vi "Verify Acoustic Calibration.vi"(0 "TSM context":T1, 5 "Cal File Path":path, 7 "Frequency - dBSPL":cluster{"Frequency (Hz)":dbl, "dB SPL":dbl}[](array[cluster])) -> (4 "Per-Site Per-FreqAmpPair dB SPL":dbl[][](array[numeric]), 15 "error out":errorcluster)   [LabVIEW 2020]
doc: "Verifies the calibration data saved in the Cal File. An array of amplitude values is obtained from the Cal file for the respective Freq-dB SPL list passed by the user. Then, a sweep is performed for Freq-Amp pair to obtain back dB SPL to calculate the Error delta (in dB SPL) which is later published to TS layer for Limit checking."
uses:
  <vilib>/NI_TestStand_SemiconductorModule/NI_TestStand_Semiconductor_Module.lvlibp/PinMap/General/SemiconductorModuleContext.ctl
  SubVIs/Per Site Sweep Data.ctl
  45f10d7d-5394-4cb1-bdbe-9d468bbd36f7.vi
  <vilib>/gmath/interp.llb/Interpolate 2D.vi
  <vilib>/gmath/interp.llb/Interpolate 2D (1d xi,yi).vi
  <vilib>/Utility/error.llb/Error Cluster From Error Code.vi
  <vilib>/NI_TestStand_SemiconductorModule/NI_TestStand_Semiconductor_Module.lvlibp/PinMap/General/Publish/PublishDataDoubleFunctionalTest.vi
  <vilib>/NI_TestStand_SemiconductorModule/NI_TestStand_Semiconductor_Module.lvlibp
panel:
  # "Test conditions ----->"
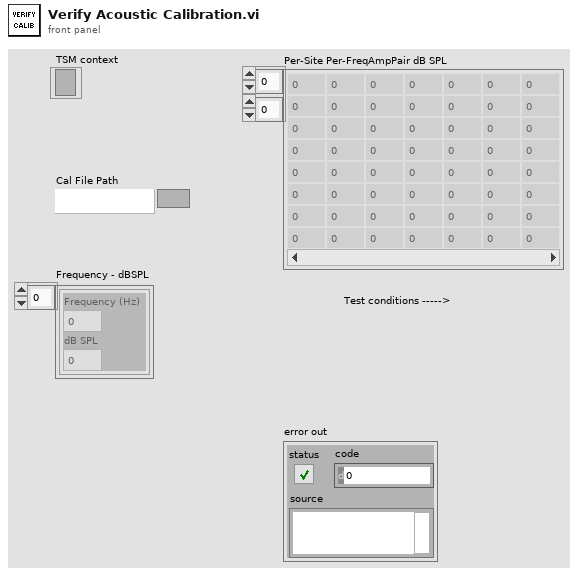
[diagram p1: front panel]
types:
  T1 = typedef "NI_TestStand_Semiconductor_Module.lvlibp/SemiconductorModuleContext.ctl" = refnum<k7>
  T2 = cluster{"TSM context":T1, "Site Numbers":i32[], "Cal File Path":path, "Sampling Rate":dbl, "Frequency - dBSPL List":cluster{"Frequency (Hz)":dbl, "dB SPL":dbl}[], "Per-Site Per-FreqAmpPair dB SPL":dbl[][]}
  T3 = typedef "Per Site Sweep Data.ctl" = cluster{"Site Number":i32, "Frequencies (Hz)":dbl[], "Amplitudes (V)":dbl[]}
  T4 = typedef "Acoustic Cal Data Cluster.ctl" = cluster{"Site Number":i32, "Serial Number":u32, "Ref Mic Sensitivity":dbl, "SPL Axis":dbl[], "Frequency Axis":dbl[], "Speaker Vp":dbl[][], "Ref Mic Cal File Data":string[][], "Speaker Vp Axis":dbl[], "SPL Measurements":dbl[][]}
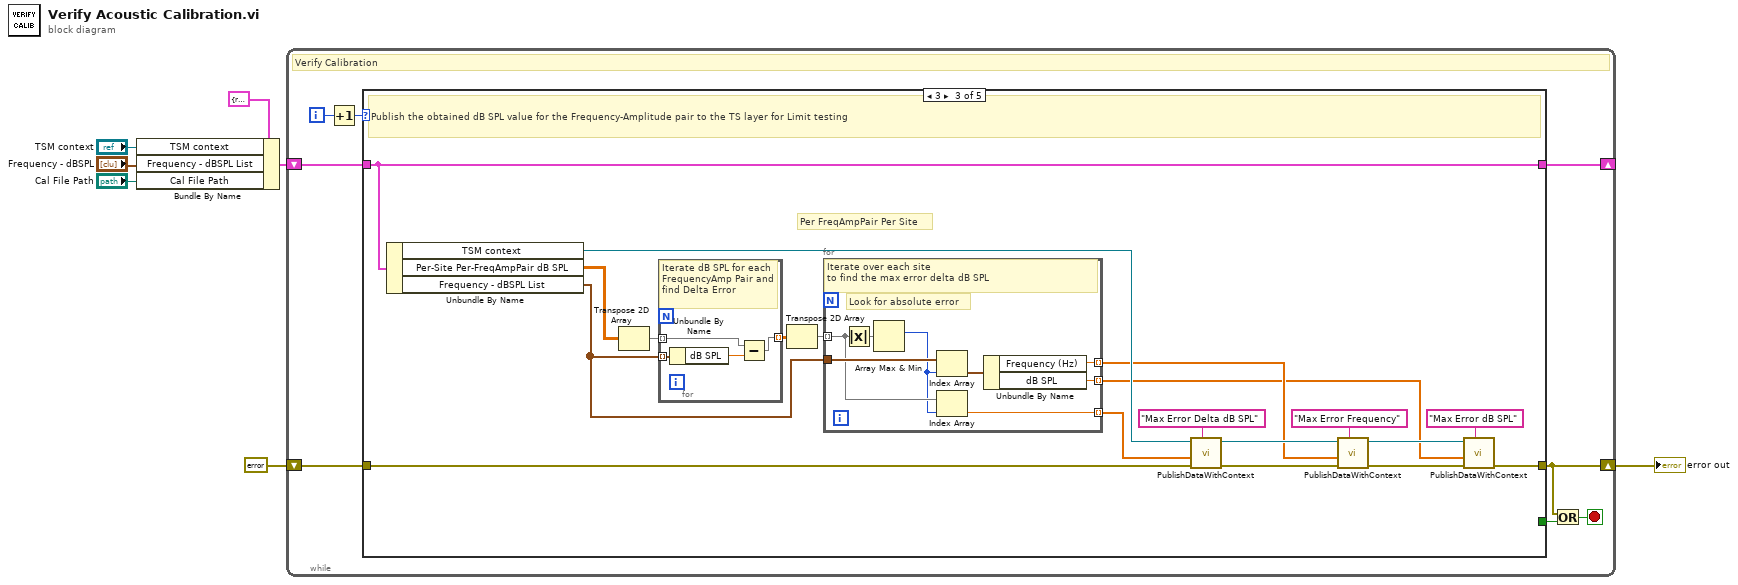
[diagram p0: block diagram]
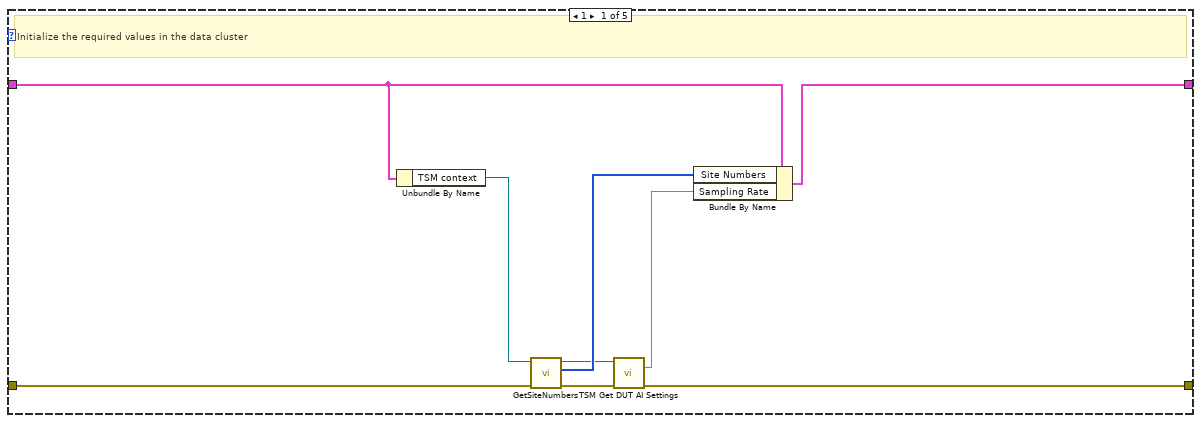
[diagram p2: hidden frame]
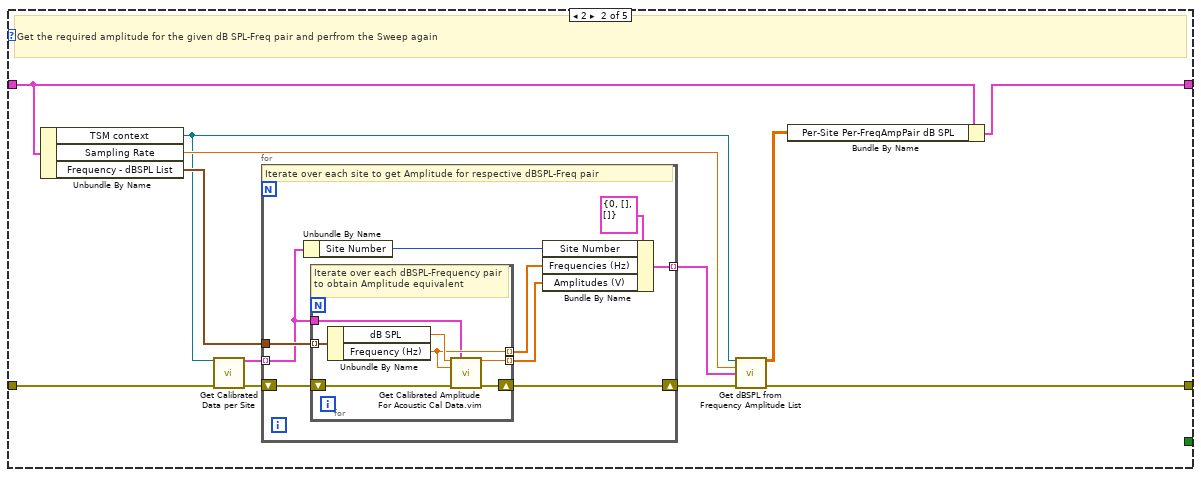
[diagram p3: hidden frame]
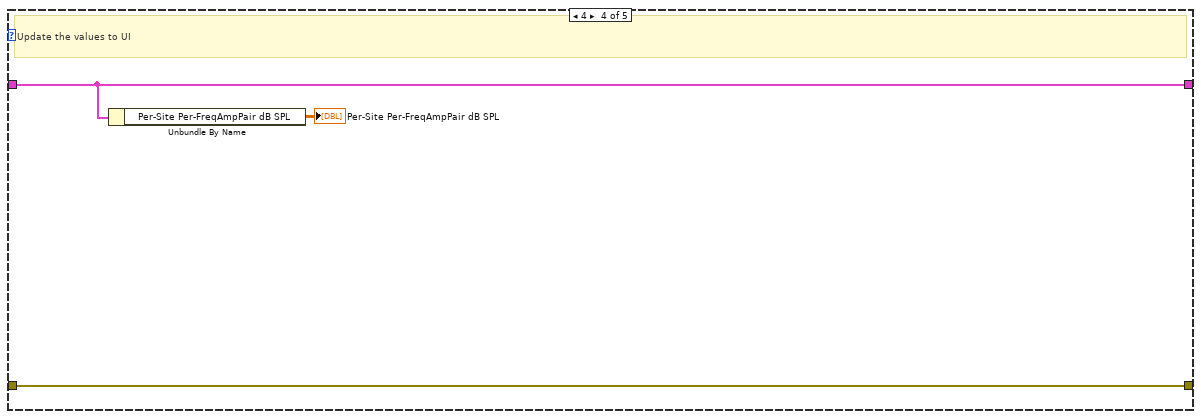
[diagram p4: hidden frame]
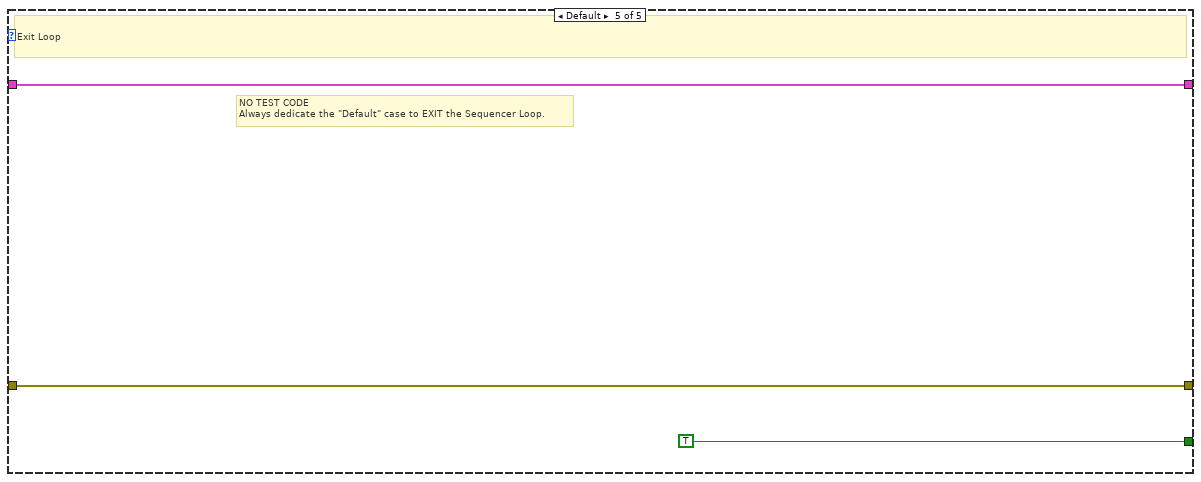
[diagram p5: hidden frame]
diagram:
  n1 = Bundle By Name(cluster=T2 {"TSM context"=refnum, "Site Numbers"=[], "Cal File Path"=path "", "Sampling Rate"=0.0, "Frequency - dBSPL List"=[], "Per-Site Per-FreqAmpPair dB SPL"=[]}, "TSM context"="TSM context", "Frequency - dBSPL List"="Frequency - dBSPL", "Cal File Path"="Cal File Path") -> (w4:T2)
  n2 = while {
    shift-right: [w8] -> w7
    shift-left: errorcluster {"status"=FALSE, "code"=0, "source"=""} ("error in") -> [w14]
    shift-right: [w10] -> _
    shift-left: w4 -> [w11]
    i -> [w15]
    stop <- w9 stop-if-true
    # "Verify Calibration"
    n3 = Increment(x=w15) -> (x+1=w13:i32)
    n4 = case shown="3" w13 {
      tunnel: [w18 w33 w53 w86 w88] -> w8
      tunnel: w14 -> [w17 w28 w65 w86 w88]
      tunnel: [_ _ _ _ TRUE] -> w12
      tunnel: w11 -> [w24 w36 w71 w85 w87]
      tunnel: [w22 w32 w71 w85 w87] -> w10
      frame 1 {
        # "Initialize the required values in the data cluster"
        n5 = Unbundle By Name(w24) -> ("TSM context"=w23:T1)
        n6 = call <vilib>:"GetSiteNumbers.vi"("error in (no error)"=w17, "Semiconductor Module Context"=w23) -> ("error out"=w16:errorcluster, "Site Numbers"=w21:i32[], "Semiconductor Module Context Out"=w20:T1)  [unwired: 6 in, 1 out]
        n7 = call "TSM Get DUT AI Settings.vi"("TSM context"=w20, "error in (no error)"=w16) -> ("Sampling Rate (Hz)"=w19:dbl, "error out"=w18:errorcluster)  [unwired: 9 in, 3 out]
        n8 = Bundle By Name(cluster=w24, "Site Numbers"=w21, "Sampling Rate"=w19) -> (w22:T2)
      }
      frame 2 {
        # "Get the required amplitude for the given dB SPL-Freq pair and perfrom the Sweep again"
        n9 = Unbundle By Name(w36) -> ("TSM context"=w27:T1, "Sampling Rate"=w35:dbl, "Frequency - dBSPL List"=w29:cluster{"Frequency (Hz)":dbl, "dB SPL":dbl}[])
        n10 = call "Get Calibrated Data per Site.vi"("TSM context"=w27, "error in (no error)"=w28) -> ("Per Site Acoustic Cal Data"=w25:T4[], "error out"=w26:errorcluster)  [unwired: 11 in, 1 out]
        n11 = for {
          shift-right: [w45] -> w34
          shift-left: w26 -> [w39]
          tunnel: w29 -> [w44]
          tunnel: [w40] -> w30 mode=indexing
          tunnel: w25 -> [w38] mode=indexing
          # "Iterate over each site to get Amplitude for respective dBSPL-Freq pair"
          n12 = Unbundle By Name(w38) -> ("Site Number"=w37:i32)
          n13 = for {
            shift-right: [w51] -> w45
            shift-left: w39 -> [w52]
            tunnel: w44 -> [w50] mode=indexing
            tunnel: [w48] -> w41 mode=indexing
            tunnel: [w47] -> w42 mode=indexing
            tunnel: w38 -> [w46]
            # "Iterate over each dBSPL-Frequency pair to obtain Amplitude equivalent"
            n14 = Unbundle By Name(w50) -> ("dB SPL"=w49:dbl, "Frequency (Hz)"=w47:dbl)
            n15 = call "Get Calibrated Amplitude For Acoustic Cal Data.vim"("dB SPL"=w49, "Acoustic Cal Data"=w46, "Frequency"=w47, "error in (no error)"=w52) -> ("Amplitude"=w48:dbl, "error out"=w51:errorcluster)  [unwired: 10 in]
          }
          n16 = Bundle By Name(cluster=T3 {"Site Number"=0, "Frequencies (Hz)"=[], "Amplitudes (V)"=[]} ("Per Site Sweep Data"), "Site Number"=w37, "Frequencies (Hz)"=w42, "Amplitudes (V)"=w41) -> (w40:T3)
        }
        n17 = call "Get dBSPL from Frequency Amplitude List.vi"("Semiconductor Module Context"=w27, "Sampling Rate"=w35, "Per Site Freq-Amp Data"=w30, "error in (no error)"=w34) -> ("Per-Site Per-FreqAmpPair dB SPL"=w31:dbl[][], "error out"=w33:errorcluster)  [unwired: 10 in]
        n18 = Bundle By Name(cluster=w36, "Per-Site Per-FreqAmpPair dB SPL"=w31) -> (w32:T2)
      }
      frame 3 {
        # "Per FreqAmpPair Per Site"
        # "Publish the obtained dB SPL value for the Frequency-Amplitude pair to the TS layer for Limit testing"
        n19 = Unbundle By Name(w71) -> ("TSM context"=w66:T1, "Per-Site Per-FreqAmpPair dB SPL"=w70:dbl[][], "Frequency - dBSPL List"=w62:cluster{"Frequency (Hz)":dbl, "dB SPL":dbl}[])
        n20 = Transpose 2D Array(2D array=w70) -> (transposed array=w69:dbl[][])
        n21 = for {
          tunnel: w69 -> [w83] mode=indexing
          tunnel: w62 -> [w81] mode=indexing
          tunnel: [w80] -> w68 mode=indexing
          # "Iterate dB SPL for each FrequencyAmp Pair and find Delta Error"
          n22 = Unbundle By Name(w81) -> ("dB SPL"=w82:dbl)
          n23 = Subtract(x=w83, y=w82) -> (x-y=w80:dbl[])
        }
        n24 = Transpose 2D Array(2D array=w68) -> (transposed array=w67:dbl[][])
        n25 = for {
          tunnel: w67 -> [w74] mode=indexing
          tunnel: [w72] -> w64 mode=indexing
          tunnel: w62 -> [w79]
          tunnel: [w77] -> w58 mode=indexing
          tunnel: [w76] -> w54 mode=indexing
          # "Look for absolute error"
          # "Iterate over each site\nto find the max error delta dB SPL"
          n26 = Absolute Value(x=w74) -> (abs(x)=w75:dbl[])
          n27 = Array Max & Min(array=w75) -> (max index (indices)=w73:i32)  [unwired: 3 out]
          n28 = Index Array(array=w79, index=w73) -> (element=w78:cluster{"Frequency (Hz)":dbl, "dB SPL":dbl})
          n29 = Index Array(array=w74, index=w73) -> (element=w72:dbl)
          n30 = Unbundle By Name(w78) -> ("Frequency (Hz)"=w77:dbl, "dB SPL"=w76:dbl)
        }
        n31 = call-poly <vilib>:"PublishDataWithContext.vi"("Published Data Id"="Max Error Delta dB SPL", "error in (no error)"=w65, "Data In"=w64, "Semiconductor Module Context"=w66) -> ("error out"=w60:errorcluster, "Semiconductor Module Context Out"=w59:T1)  [unwired: 6 in]
        n32 = call-poly <vilib>:"PublishDataWithContext.vi"("Published Data Id"="Max Error Frequency", "error in (no error)"=w60, "Data In"=w58, "Semiconductor Module Context"=w59) -> ("error out"=w56:errorcluster, "Semiconductor Module Context Out"=w55:T1)  [unwired: 6 in]
        n33 = call-poly <vilib>:"PublishDataWithContext.vi"("Published Data Id"="Max Error dB SPL", "error in (no error)"=w56, "Data In"=w54, "Semiconductor Module Context"=w55) -> ("error out"=w53:errorcluster)  [unwired: 6 in, 1 out]
      }
      frame 4 {
        # "Update the values to UI"
        n34 = Unbundle By Name(w85) -> ("Per-Site Per-FreqAmpPair dB SPL"=→"Per-Site Per-FreqAmpPair dB SPL":dbl[][])
      }
      frame Default {
        # "NO TEST CODE\nAlways dedicate the \"Default\" case to EXIT the Sequencer Loop."
        # "Exit Loop"
      }
    }
    n35 = Or(x=w8, y=w12) -> (x .or. y?=w9:bool)
  }
  "error out" <- w7
